vi "while_factorial.vi"(1 "Number":dbl) -> (0 "Factorial":dbl)   [LabVIEW 2023]
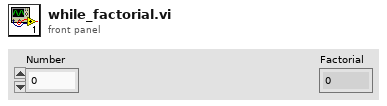
[diagram p1: front panel]
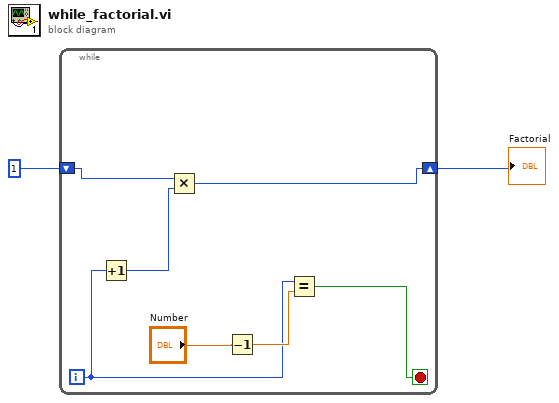
[diagram p0: block diagram]
diagram:
  n1 = while {
    shift-right: [w6] -> w2
    shift-left: 1 -> [w5]
    i -> [w3]
    stop <- w7 stop-if-true
    n2 = Increment(x=w3) -> (x+1=w4:i32)
    n3 = Multiply(x=w5, y=w4) -> (x*y=w6:i32)
    n4 = Decrement(x="Number") -> (x-1=w8:dbl)
    n5 = Equal?(x=w3, y=w8) -> (x = y?=w7:bool)
  }
  "Factorial" <- w2
